vi "Finish.vi"   [LabVIEW 2018]
doc: "This VI is called just before exiting. It is expected to close I/O refnum, save collected data, etc."
uses:
  <vilib>/Rock Robotics/WPI/Utilities/WPI_GetSetVariantRefNum.vi
types:
  T1 = typedef "WPI_MotorControlDeviceRef.ctl" = cluster{"DeviceStatus":errorcluster, "Type":T2, "PWM":cluster{"PWM Channel":T3, "DeadBand":T4}, "CAN":cluster{"Device Number":u8, "SetOutput VI Ref":variant, "GetOutput VI Ref":variant, "Enable VI Ref":variant, "Disable VI Ref":variant, "Data":variant}, "Invert":bool, "DIO PWM":cluster{"PWM \"Enable\" Channel":T3, "DIOChannel":T5, "PWM Rate":dbl}}
  T2 = typedef "WPI_MotorControlType.ctl" = enum16{"PWM", "CAN", "DIO PWM"}
  T3 = typedef "FPGA_DIOPWMChannel.ctl" = enum8{"PWM 0", "PWM 1", "PWM 2", "PWM 3", "PWM 4", "PWM 5", "PWM 6", "PWM 7", "PWM 8", "PWM 9", "PWM MXP 0", "PWM MXP 1", "PWM MXP 2", "PWM MXP 3", "PWM MXP 4", "PWM MXP 5", "PWM MXP 6", "PWM MXP 7", "PWM MXP 8", "PWM MXP 9", "Invalid"}
  T4 = typedef "WPI_PWMDeadband.ctl" = cluster{"Name":string, "maxPositivePwm":i32, "minPositivePwm":i32, "centerPwm":i32, "maxNegativePwm":i32, "minNegativePwm":i32, "angularRange":u16}
  T5 = typedef "FPGA_DIOChannel.ctl" = enum8{"DIO 0", "DIO 1", "DIO 2", "DIO 3", "DIO 4", "DIO 5", "DIO 6", "DIO 7", "DIO 8", "DIO 9", "DIO MXP 0", "DIO MXP 1", "DIO MXP 2", "DIO MXP 3", "DIO MXP 4", "DIO MXP 5", "DIO MXP 6", "DIO MXP 7", "DIO MXP 8", "DIO MXP 9", "DIO MXP 10", "DIO MXP 11", "DIO MXP 12", "DIO MXP 13", "DIO MXP 14", "DIO MXP 15", "SPI Port CS1", "SPI Port CS2", "SPI Port CS3", "SPI Port MISO", "SPI Port MOSI", "Invalid"}
  T6 = typedef "WPI_RobotDriveDevRef.ctl" = cluster{"DevStatus":errorcluster, "Motors[]":T1[], "Square Inputs":bool, "Max Output":dbl}
  T7 = typedef "WPI_CompressorDevRef.ctl" = cluster{"DevStatus":errorcluster, "Pneumatics Control Module":u8}
  T8 = typedef "WPI_SolenoidDevRef.ctl" = cluster{"DevStatus":errorcluster, "Pneumatics Control Module":u8, "Forward Solenoid Channel":T9, "Reverse Solenoid Channel":T9}
  T9 = typedef "WPI_SolenoidChannel.ctl" = enum8{"Solenoid 0", "Solenoid 1", "Solenoid 2", "Solenoid 3", "Solenoid 4", "Solenoid 5", "Solenoid 6", "Solenoid 7", "Invalid"}
  T10 = typedef "WPI_JoystickDevRef.ctl" = cluster{"Device":T11}
  T11 = typedef "WPI_JoystickDeviceEnum.ctl" = enum16{"USB 0", "USB 1", "USB 2", "USB 3", "USB 4", "USB 5"}
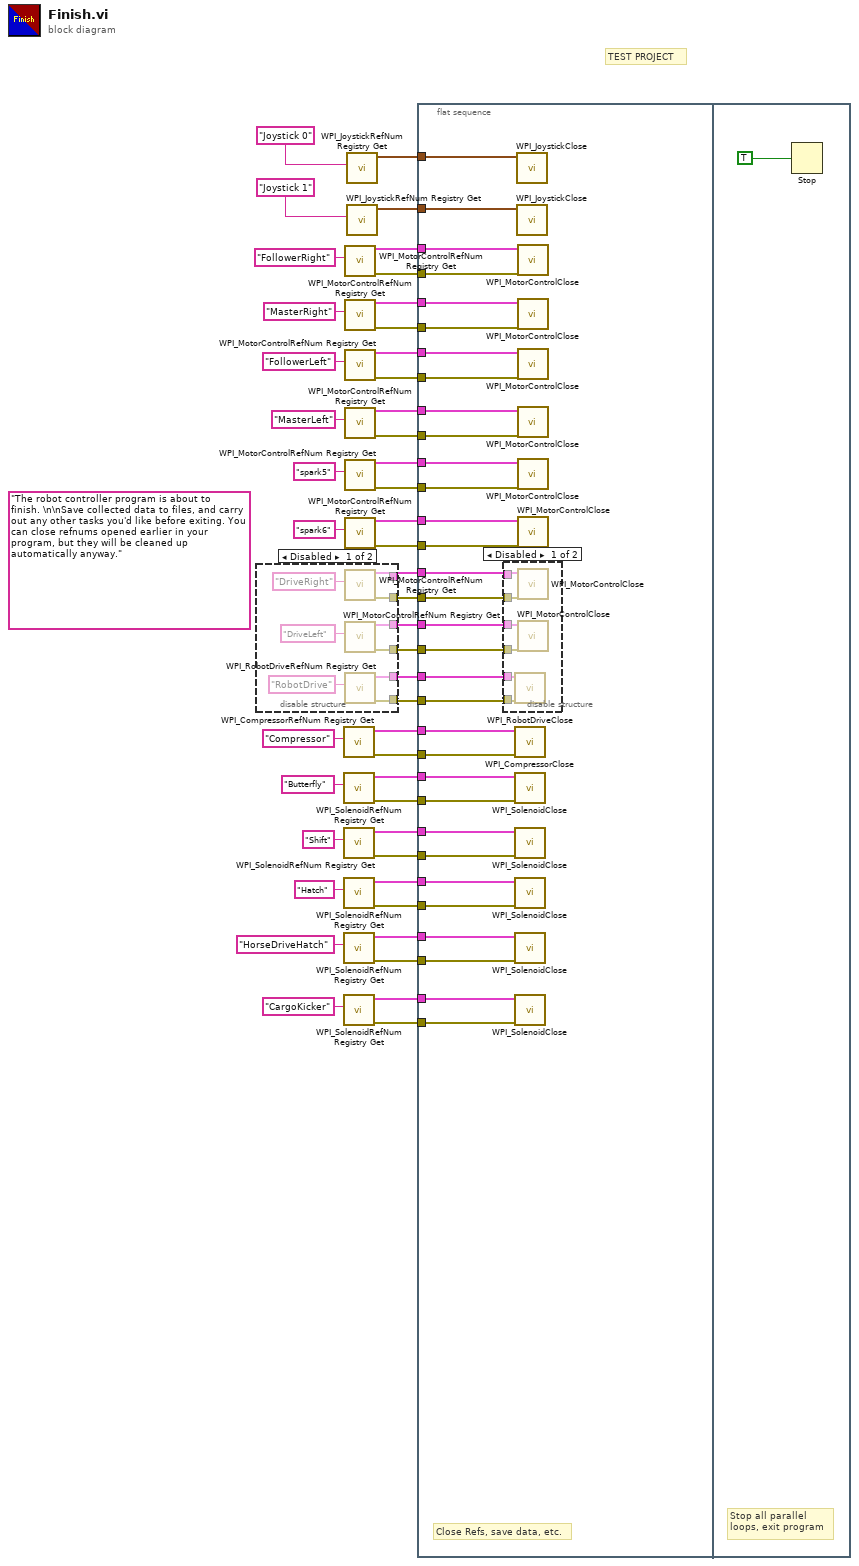
[diagram p0: block diagram]
diagram:
  (unwired) "The robot controller program is about to finish. \n\nSave collected data to files, and carry out any other tasks you'd like before exiting. You can close refnums opened earlier in your program, but they will be cleaned up automatically anyway."
  # "TEST PROJECT"
  n1 = disable-structure shown="Disabled" {
    disable-tunnel: [w54 _] -> w26
    disable-tunnel: [w53 _] -> w25
    disable-tunnel: [w52 _] -> w24
    disable-tunnel: [w51 _] -> w23
    disable-tunnel: [w49 _] -> w22
    disable-tunnel: [w48 _] -> w21
    frame Disabled {
      n2 = call <vilib>:"WPI_MotorControlRefNum Registry Get.vi"("refnum name"="DriveRight") -> ("error out"=w51:errorcluster, "MotorControlDevRef"=w52:T1)  [unwired: 9 in]
      n3 = call <vilib>:"WPI_MotorControlRefNum Registry Get.vi"("refnum name"="DriveLeft") -> ("error out"=w54:errorcluster, "MotorControlDevRef"=w53:T1)  [unwired: 9 in]
      n4 = call <vilib>:"WPI_RobotDriveRefNum Registry Get.vi"("refnum name"="RobotDrive") -> ("error out"=w48:errorcluster, "RobotDriveDevRef"=w49:T6)  [unwired: 9 in]
    }
    frame Enabled {
    }
  }
  n5 = call <vilib>:"WPI_CompressorRefNum Registry Get.vi"("refnum name"="Compressor") -> ("error out"=w18:errorcluster, "CompressorDevRef"=w19:T7)  [unwired: 9 in]
  n6 = call <vilib>:"WPI_SolenoidRefNum Registry Get.vi"("refnum name"="Butterfly") -> ("error out"=w16:errorcluster, "SolenoidDevRef"=w17:T8)  [unwired: 9 in]
  n7 = call <vilib>:"WPI_SolenoidRefNum Registry Get.vi"("refnum name"="Shift") -> ("error out"=w13:errorcluster, "SolenoidDevRef"=w12:T8)  [unwired: 9 in]
  n8 = call <vilib>:"WPI_SolenoidRefNum Registry Get.vi"("refnum name"="Hatch") -> ("error out"=w7:errorcluster, "SolenoidDevRef"=w6:T8)  [unwired: 9 in]
  n9 = call <vilib>:"WPI_SolenoidRefNum Registry Get.vi"("refnum name"="HorseDriveHatch") -> ("error out"=w10:errorcluster, "SolenoidDevRef"=w11:T8)  [unwired: 9 in]
  n10 = call <vilib>:"WPI_SolenoidRefNum Registry Get.vi"("refnum name"="CargoKicker") -> ("error out"=w4:errorcluster, "SolenoidDevRef"=w3:T8)  [unwired: 9 in]
  n11 = call <vilib>:"WPI_MotorControlRefNum Registry Get.vi"("refnum name"="FollowerRight") -> ("error out"=w43:errorcluster, "MotorControlDevRef"=w44:T1)  [unwired: 9 in]
  n12 = call <vilib>:"WPI_MotorControlRefNum Registry Get.vi"("refnum name"="MasterRight") -> ("error out"=w40:errorcluster, "MotorControlDevRef"=w39:T1)  [unwired: 9 in]
  n13 = call <vilib>:"WPI_MotorControlRefNum Registry Get.vi"("refnum name"="FollowerLeft") -> ("error out"=w37:errorcluster, "MotorControlDevRef"=w38:T1)  [unwired: 9 in]
  n14 = call <vilib>:"WPI_MotorControlRefNum Registry Get.vi"("refnum name"="MasterLeft") -> ("error out"=w34:errorcluster, "MotorControlDevRef"=w33:T1)  [unwired: 9 in]
  n15 = call <vilib>:"WPI_MotorControlRefNum Registry Get.vi"("refnum name"="spark5") -> ("error out"=w31:errorcluster, "MotorControlDevRef"=w32:T1)  [unwired: 9 in]
  n16 = call <vilib>:"WPI_MotorControlRefNum Registry Get.vi"("refnum name"="spark6") -> ("error out"=w28:errorcluster, "MotorControlDevRef"=w27:T1)  [unwired: 9 in]
  n17 = call <vilib>:"WPI_JoystickRefNum Registry Get.vi"("refnum name"="Joystick 0") -> ("JoystickDevRef"=w45:T10)  [unwired: 1 in, 9 out]
  n18 = call <vilib>:"WPI_JoystickRefNum Registry Get.vi"("refnum name"="Joystick 1") -> ("JoystickDevRef"=w2:T10)  [unwired: 1 in, 9 out]
  n19 = flat-sequence {
    tunnel: w45 -> [w87]
    tunnel: w44 -> [w86]
    tunnel: w43 -> [w85]
    tunnel: w39 -> [w83]
    tunnel: w40 -> [w84]
    tunnel: w38 -> [w82]
    tunnel: w37 -> [w81]
    tunnel: w33 -> [w79]
    tunnel: w34 -> [w80]
    tunnel: w32 -> [w78]
    tunnel: w31 -> [w77]
    tunnel: w27 -> [w75]
    tunnel: w28 -> [w76]
    tunnel: w24 -> [w72]
    tunnel: w23 -> [w71]
    tunnel: w25 -> [w73]
    tunnel: w26 -> [w74]
    tunnel: w22 -> [w70]
    tunnel: w21 -> [w69]
    tunnel: w19 -> [w68]
    tunnel: w18 -> [w67]
    tunnel: w17 -> [w66]
    tunnel: w16 -> [w65]
    tunnel: w12 -> [w63]
    tunnel: w13 -> [w64]
    tunnel: w6 -> [w59]
    tunnel: w7 -> [w60]
    tunnel: w11 -> [w62]
    tunnel: w10 -> [w61]
    tunnel: w3 -> [w57]
    tunnel: w4 -> [w58]
    tunnel: w2 -> [w56]
    frame #0 {
      # "Close Refs, save data, etc."
      n20 = disable-structure shown="Disabled" {
        disable-tunnel: w74 -> [w93 _]
        disable-tunnel: w73 -> [w92 _]
        disable-tunnel: w72 -> [w91 _]
        disable-tunnel: w71 -> [w90 _]
        disable-tunnel: w70 -> [w89 _]
        disable-tunnel: w69 -> [w88 _]
        frame Disabled {
          n21 = call <vilib>:"WPI_RobotDriveClose.vi"("error in (no error)"=w88, "RobotDriveDevRef"=w89) -> ()  [unwired: 9 in, 1 out]
          n22 = call <vilib>:"WPI_MotorControlClose.vi"("error in"=w90, "MotorControlDevRef"=w91) -> ()  [unwired: 9 in, 1 out]
          n23 = call <vilib>:"WPI_MotorControlClose.vi"("error in"=w93, "MotorControlDevRef"=w92) -> ()  [unwired: 9 in, 1 out]
        }
        frame Enabled {
        }
      }
      n24 = call <vilib>:"WPI_CompressorClose.vi"("error in (no error)"=w67, "CompressorDevRef"=w68) -> ()  [unwired: 9 in, 1 out]
      n25 = call <vilib>:"WPI_SolenoidClose.vi"("error in (no error)"=w65, "SolenoidDevRef"=w66) -> ()  [unwired: 9 in, 1 out]
      n26 = call <vilib>:"WPI_SolenoidClose.vi"("error in (no error)"=w64, "SolenoidDevRef"=w63) -> ()  [unwired: 9 in, 1 out]
      n27 = call <vilib>:"WPI_SolenoidClose.vi"("error in (no error)"=w60, "SolenoidDevRef"=w59) -> ()  [unwired: 9 in, 1 out]
      n28 = call <vilib>:"WPI_SolenoidClose.vi"("error in (no error)"=w61, "SolenoidDevRef"=w62) -> ()  [unwired: 9 in, 1 out]
      n29 = call <vilib>:"WPI_SolenoidClose.vi"("error in (no error)"=w58, "SolenoidDevRef"=w57) -> ()  [unwired: 9 in, 1 out]
      n30 = call <vilib>:"WPI_JoystickClose.vi"("JoystickDevRef"=w87) -> ()  [unwired: 11 out]
      n31 = call <vilib>:"WPI_JoystickClose.vi"("JoystickDevRef"=w56) -> ()  [unwired: 11 out]
      n32 = call <vilib>:"WPI_MotorControlClose.vi"("error in"=w85, "MotorControlDevRef"=w86) -> ()  [unwired: 9 in, 1 out]
      n33 = call <vilib>:"WPI_MotorControlClose.vi"("error in"=w84, "MotorControlDevRef"=w83) -> ()  [unwired: 9 in, 1 out]
      n34 = call <vilib>:"WPI_MotorControlClose.vi"("error in"=w81, "MotorControlDevRef"=w82) -> ()  [unwired: 9 in, 1 out]
      n35 = call <vilib>:"WPI_MotorControlClose.vi"("error in"=w80, "MotorControlDevRef"=w79) -> ()  [unwired: 9 in, 1 out]
      n36 = call <vilib>:"WPI_MotorControlClose.vi"("error in"=w77, "MotorControlDevRef"=w78) -> ()  [unwired: 9 in, 1 out]
      n37 = call <vilib>:"WPI_MotorControlClose.vi"("error in"=w76, "MotorControlDevRef"=w75) -> ()  [unwired: 9 in, 1 out]
    }
    frame #1 {
      # "Stop all parallel\nloops, exit program"
      n38 = Stop(stop? (T)=TRUE ("Quit")) -> ()
    }
  }
